vi "Reactor_Coolant_Pump_Motor_Speed_Loop.vi"(0 "SI600.lvclass in":refnum<class "SI600.lvclass">, 1 "3 JEB CS951 XQ01":dbl, 2 "3 JEB CS952 XQ01":dbl, 3 "3 JEB CS953 XQ01":dbl, 4 "3 JEB CS954 XQ01":dbl, 6 "Loop":enum16{"LOOP10", "LOOP20", "LOOP30", "LOOP40"}(ring), 7 "error in (no error)":errorcluster) -> (20 "SI600.lvclass out":refnum<class "SI600.lvclass">, 21 "RCP speed Loop Output":dbl, 22 "3 JEB CS951":dbl, 23 "3 JEB CS952":dbl, 24 "3 JEB CS953":dbl, 25 "3 JEB CS954":dbl, 27 "error IO":errorcluster)   [LabVIEW 2022 SP3, in "SI600.lvclass"]
uses:
  SI600.lvclass
  SI600.lvclass/SI600.ctl
panel:
  # "SI600"
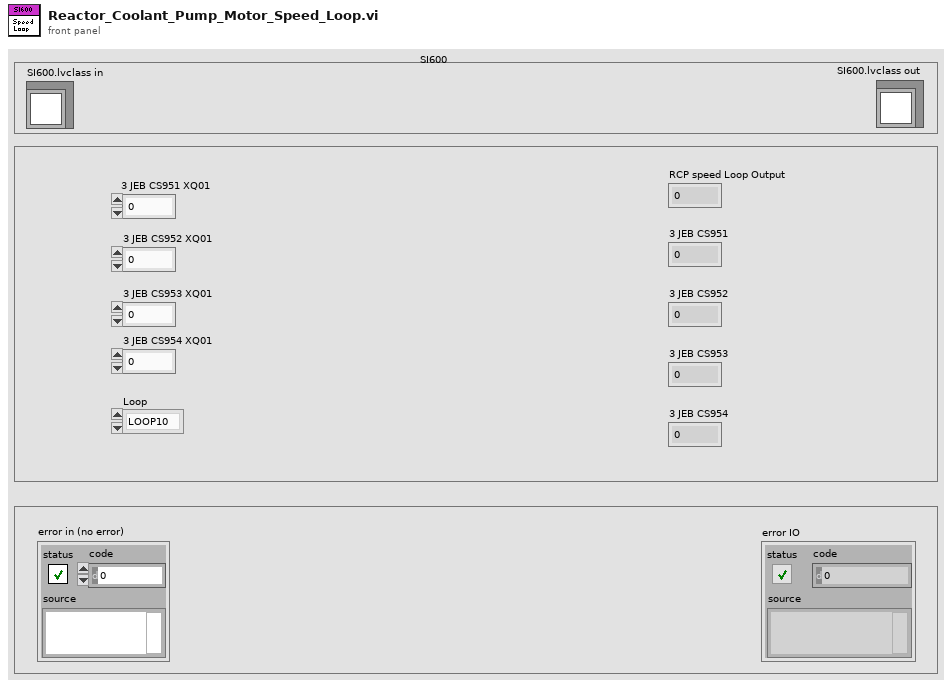
[diagram p1: front panel]
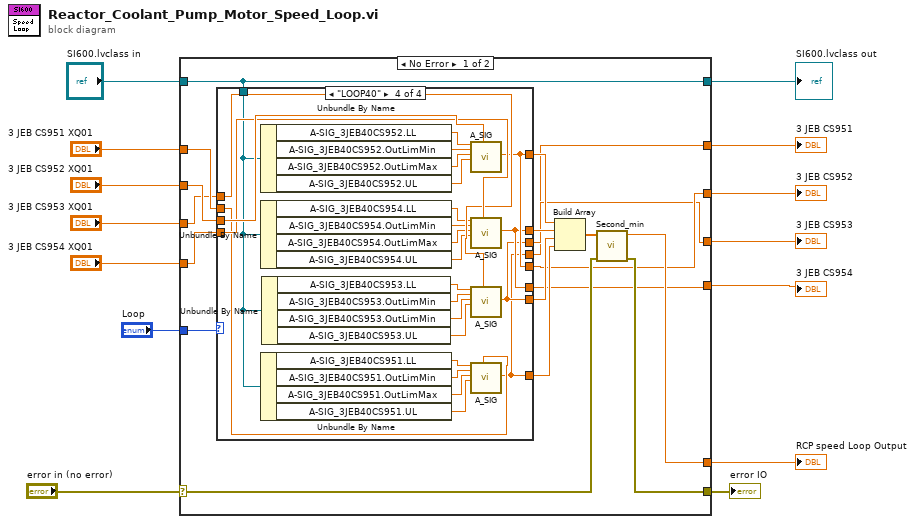
[diagram p0: block diagram]
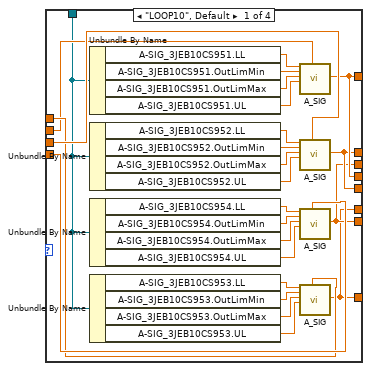
[diagram p2: hidden frame]
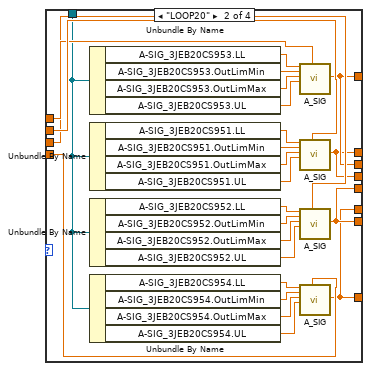
[diagram p3: hidden frame]
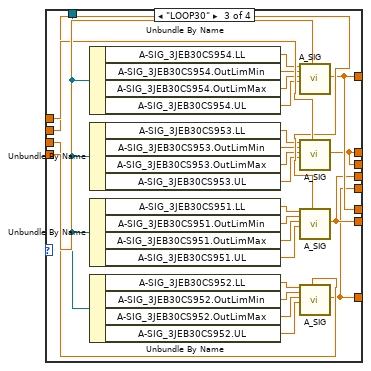
[diagram p4: hidden frame]
diagram:
  n1 = case shown="No Error" "error in (no error)" {
    selector: "error in (no error)" -> [w29 w134]
    tunnel: "SI600.lvclass in" -> [w15 w133]
    tunnel: [w15 w133] -> w11
    tunnel: [w31 _] -> w13
    tunnel: [w28 w134] -> w12
    tunnel: "Loop" -> [w30 _]
    tunnel: "3 JEB CS951 XQ01" -> [w23 _]
    tunnel: "3 JEB CS952 XQ01" -> [w22 _]
    tunnel: "3 JEB CS954 XQ01" -> [w21 _]
    tunnel: "3 JEB CS953 XQ01" -> [w20 _]
    tunnel: [w19 _] -> w4
    tunnel: [w18 _] -> w3
    tunnel: [w17 _] -> w2
    tunnel: [w16 _] -> w1
    frame No Error {
      n2 = case shown="\"LOOP40\"" w30 {
        tunnel: [w34 w59 w84 w109] -> w27
        tunnel: [w35 w60 w85 w110] -> w26
        tunnel: [w36 w61 w86 w111] -> w25
        tunnel: [w37 w62 w87 w112] -> w24
        tunnel: w23 -> [w38 w82 w105 w129]
        tunnel: w22 -> [w41 w80 w104 w132]
        tunnel: w21 -> [w40 w79 w107 w131]
        tunnel: w20 -> [w39 w81 w106 w130]
        tunnel: [w36 w60 w84 w112] -> w19
        tunnel: [w34 w59 w87 w111] -> w18
        tunnel: [w35 w62 w86 w110] -> w17
        tunnel: [w37 w61 w85 w109] -> w16
        tunnel: w15 -> [w33 w58 w83 w108]
        frame "LOOP10", Default {
          n3 = Unbundle By Name(w33) -> ("A-SIG_3JEB10CS951.LL"=w57:dbl, "A-SIG_3JEB10CS951.OutLimMin"=w56:dbl, "A-SIG_3JEB10CS951.OutLimMax"=w55:dbl, "A-SIG_3JEB10CS951.UL"=w54:dbl)
          n4 = Unbundle By Name(w33) -> ("A-SIG_3JEB10CS952.LL"=w53:dbl, "A-SIG_3JEB10CS952.OutLimMin"=w52:dbl, "A-SIG_3JEB10CS952.OutLimMax"=w51:dbl, "A-SIG_3JEB10CS952.UL"=w50:dbl)
          n5 = Unbundle By Name(w33) -> ("A-SIG_3JEB10CS954.LL"=w49:dbl, "A-SIG_3JEB10CS954.OutLimMin"=w48:dbl, "A-SIG_3JEB10CS954.OutLimMax"=w47:dbl, "A-SIG_3JEB10CS954.UL"=w46:dbl)
          n6 = Unbundle By Name(w33) -> ("A-SIG_3JEB10CS953.LL"=w45:dbl, "A-SIG_3JEB10CS953.OutLimMin"=w44:dbl, "A-SIG_3JEB10CS953.OutLimMax"=w43:dbl, "A-SIG_3JEB10CS953.UL"=w42:dbl)
          n7 = call "A_SIG.vi"("LL"=w57, "OutLimMin"=w56, "OutLimMax"=w55, "UL"=w54, "Input"=w38) -> ("A_SIG_out"=w37:dbl)  [unwired: 13 in, 1 out]
          n8 = call "A_SIG.vi"("LL"=w53, "OutLimMin"=w52, "OutLimMax"=w51, "UL"=w50, "Input"=w41) -> ("A_SIG_out"=w36:dbl)  [unwired: 13 in, 1 out]
          n9 = call "A_SIG.vi"("LL"=w49, "OutLimMin"=w48, "OutLimMax"=w47, "UL"=w46, "Input"=w40) -> ("A_SIG_out"=w35:dbl)  [unwired: 13 in, 1 out]
          n10 = call "A_SIG.vi"("LL"=w45, "OutLimMin"=w44, "OutLimMax"=w43, "UL"=w42, "Input"=w39) -> ("A_SIG_out"=w34:dbl)  [unwired: 13 in, 1 out]
        }
        frame "LOOP20" {
          n11 = Unbundle By Name(w58) -> ("A-SIG_3JEB20CS953.LL"=w78:dbl, "A-SIG_3JEB20CS953.OutLimMin"=w77:dbl, "A-SIG_3JEB20CS953.OutLimMax"=w76:dbl, "A-SIG_3JEB20CS953.UL"=w75:dbl)
          n12 = Unbundle By Name(w58) -> ("A-SIG_3JEB20CS951.LL"=w74:dbl, "A-SIG_3JEB20CS951.OutLimMin"=w73:dbl, "A-SIG_3JEB20CS951.OutLimMax"=w72:dbl, "A-SIG_3JEB20CS951.UL"=w71:dbl)
          n13 = Unbundle By Name(w58) -> ("A-SIG_3JEB20CS952.LL"=w70:dbl, "A-SIG_3JEB20CS952.OutLimMin"=w69:dbl, "A-SIG_3JEB20CS952.OutLimMax"=w68:dbl, "A-SIG_3JEB20CS952.UL"=w67:dbl)
          n14 = Unbundle By Name(w58) -> ("A-SIG_3JEB20CS954.LL"=w66:dbl, "A-SIG_3JEB20CS954.OutLimMin"=w65:dbl, "A-SIG_3JEB20CS954.OutLimMax"=w64:dbl, "A-SIG_3JEB20CS954.UL"=w63:dbl)
          n15 = call "A_SIG.vi"("LL"=w78, "OutLimMin"=w77, "OutLimMax"=w76, "UL"=w75, "Input"=w81) -> ("A_SIG_out"=w62:dbl)  [unwired: 13 in, 1 out]
          n16 = call "A_SIG.vi"("LL"=w74, "OutLimMin"=w73, "OutLimMax"=w72, "UL"=w71, "Input"=w82) -> ("A_SIG_out"=w61:dbl)  [unwired: 13 in, 1 out]
          n17 = call "A_SIG.vi"("LL"=w70, "OutLimMin"=w69, "OutLimMax"=w68, "UL"=w67, "Input"=w80) -> ("A_SIG_out"=w60:dbl)  [unwired: 13 in, 1 out]
          n18 = call "A_SIG.vi"("LL"=w66, "OutLimMin"=w65, "OutLimMax"=w64, "UL"=w63, "Input"=w79) -> ("A_SIG_out"=w59:dbl)  [unwired: 13 in, 1 out]
        }
        frame "LOOP30" {
          n19 = Unbundle By Name(w83) -> ("A-SIG_3JEB30CS954.LL"=w103:dbl, "A-SIG_3JEB30CS954.OutLimMin"=w102:dbl, "A-SIG_3JEB30CS954.OutLimMax"=w101:dbl, "A-SIG_3JEB30CS954.UL"=w100:dbl)
          n20 = Unbundle By Name(w83) -> ("A-SIG_3JEB30CS953.LL"=w99:dbl, "A-SIG_3JEB30CS953.OutLimMin"=w98:dbl, "A-SIG_3JEB30CS953.OutLimMax"=w97:dbl, "A-SIG_3JEB30CS953.UL"=w96:dbl)
          n21 = Unbundle By Name(w83) -> ("A-SIG_3JEB30CS951.LL"=w95:dbl, "A-SIG_3JEB30CS951.OutLimMin"=w94:dbl, "A-SIG_3JEB30CS951.OutLimMax"=w93:dbl, "A-SIG_3JEB30CS951.UL"=w92:dbl)
          n22 = Unbundle By Name(w83) -> ("A-SIG_3JEB30CS952.LL"=w91:dbl, "A-SIG_3JEB30CS952.OutLimMin"=w90:dbl, "A-SIG_3JEB30CS952.OutLimMax"=w89:dbl, "A-SIG_3JEB30CS952.UL"=w88:dbl)
          n23 = call "A_SIG.vi"("LL"=w103, "OutLimMin"=w102, "OutLimMax"=w101, "UL"=w100, "Input"=w107) -> ("A_SIG_out"=w87:dbl)  [unwired: 13 in, 1 out]
          n24 = call "A_SIG.vi"("LL"=w99, "OutLimMin"=w98, "OutLimMax"=w97, "UL"=w96, "Input"=w106) -> ("A_SIG_out"=w86:dbl)  [unwired: 13 in, 1 out]
          n25 = call "A_SIG.vi"("LL"=w95, "OutLimMin"=w94, "OutLimMax"=w93, "UL"=w92, "Input"=w105) -> ("A_SIG_out"=w85:dbl)  [unwired: 13 in, 1 out]
          n26 = call "A_SIG.vi"("LL"=w91, "OutLimMin"=w90, "OutLimMax"=w89, "UL"=w88, "Input"=w104) -> ("A_SIG_out"=w84:dbl)  [unwired: 13 in, 1 out]
        }
        frame "LOOP40" {
          n27 = Unbundle By Name(w108) -> ("A-SIG_3JEB40CS952.LL"=w128:dbl, "A-SIG_3JEB40CS952.OutLimMin"=w127:dbl, "A-SIG_3JEB40CS952.OutLimMax"=w126:dbl, "A-SIG_3JEB40CS952.UL"=w125:dbl)
          n28 = Unbundle By Name(w108) -> ("A-SIG_3JEB40CS954.LL"=w124:dbl, "A-SIG_3JEB40CS954.OutLimMin"=w123:dbl, "A-SIG_3JEB40CS954.OutLimMax"=w122:dbl, "A-SIG_3JEB40CS954.UL"=w121:dbl)
          n29 = Unbundle By Name(w108) -> ("A-SIG_3JEB40CS951.LL"=w116:dbl, "A-SIG_3JEB40CS951.OutLimMin"=w115:dbl, "A-SIG_3JEB40CS951.OutLimMax"=w114:dbl, "A-SIG_3JEB40CS951.UL"=w113:dbl)
          n30 = Unbundle By Name(w108) -> ("A-SIG_3JEB40CS953.LL"=w120:dbl, "A-SIG_3JEB40CS953.OutLimMin"=w119:dbl, "A-SIG_3JEB40CS953.OutLimMin"=w118:dbl, "A-SIG_3JEB40CS953.UL"=w117:dbl)
          n31 = call "A_SIG.vi"("LL"=w128, "OutLimMin"=w127, "OutLimMax"=w126, "UL"=w125, "Input"=w132) -> ("A_SIG_out"=w112:dbl)  [unwired: 13 in, 1 out]
          n32 = call "A_SIG.vi"("LL"=w124, "OutLimMin"=w123, "OutLimMax"=w122, "UL"=w121, "Input"=w131) -> ("A_SIG_out"=w111:dbl)  [unwired: 13 in, 1 out]
          n33 = call "A_SIG.vi"("LL"=w120, "OutLimMin"=w119, "OutLimMax"=w118, "UL"=w117, "Input"=w130) -> ("A_SIG_out"=w110:dbl)  [unwired: 13 in, 1 out]
          n34 = call "A_SIG.vi"("LL"=w116, "OutLimMin"=w115, "OutLimMax"=w114, "UL"=w113, "Input"=w129) -> ("A_SIG_out"=w109:dbl)  [unwired: 13 in, 1 out]
        }
      }
      n35 = Build Array(w24, w25, w26, w27) -> (w32:dbl[])
      n36 = call "Second_min.vi"("error in (no error)"=w29, "Array"=w32) -> ("error IO"=w28:errorcluster, "output"=w31:dbl)  [unwired: 8 in]
    }
    frame Error {
    }
  }
  "3 JEB CS951" <- w1
  "3 JEB CS952" <- w4
  "3 JEB CS953" <- w2
  "3 JEB CS954" <- w3
  "RCP speed Loop Output" <- w13
  "error IO" <- w12
  "SI600.lvclass out" <- w11
